vi "SPI FPGA.vi"   [LabVIEW 2014]
uses:
  SPIBus0/IO Node Logic Template_SPIBus0.lvlib
  <vilib>/rvi/DataTransferAndStorage/Container/XNode/niFpgaContainer.xnode
  <vilib>/rvi/interface/RandomDataEmulation/nirviRandomDataFpgaReadWriteTemplate.vi
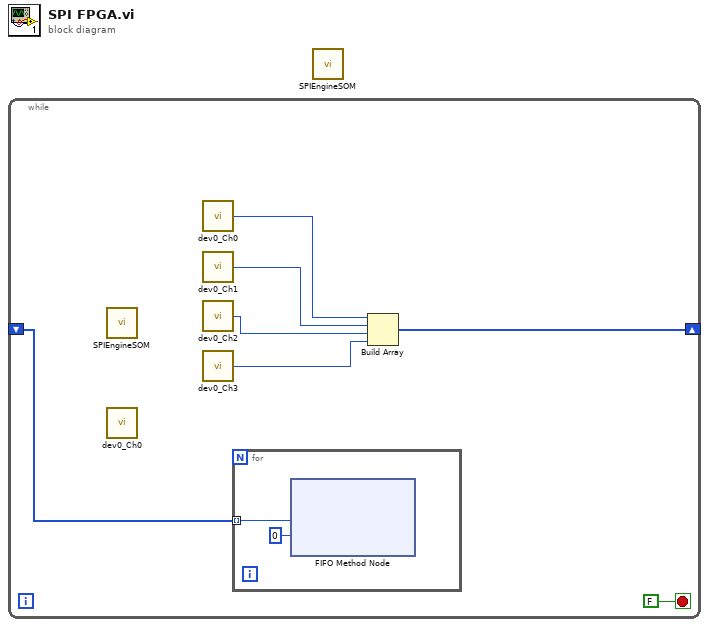
[diagram p0: block diagram]
diagram:
  n1 = while {
    shift-right: [w7] -> _
    shift-left: _ -> [w6]
    stop <- FALSE stop-if-true
    n2 = call "dev0_Ch0.vi"() -> ("Received Data"=w4:u64)  [unwired: 15 in]
    n3 = call "dev0_Ch1.vi"() -> ("Received Data"=w3:u64)  [unwired: 15 in]
    n4 = call "dev0_Ch2.vi"() -> ("Received Data"=w2:u64)  [unwired: 15 in]
    n5 = call "dev0_Ch3.vi"() -> ("Received Data"=w1:u64)  [unwired: 15 in]
    n6 = for {
      tunnel: w6 -> [w9] mode=indexing
      n7 = xnode ("FIFO Method Node")("Element"=w9, "Timeout"=0) -> ()  [unwired: 1 in, 2 out]
    }
    n8 = Build Array(w4, w3, w2, w1) -> (w7:u64[])
  }
  n9 = call "SPIEngineSOM.vi"() -> ()  [unwired: 12 in]
  n10 = call "dev0_Ch0.vi"() -> ()  [unwired: 15 in, 1 out]
  n11 = call "SPIEngineSOM.vi"() -> ()  [unwired: 12 in]
